vi "Address2ControlPoint.vi"(10 "Address":string) -> (1 "Contol\nPoint\nSuffix":T1, 3 "ControlPoint":string)   [LabVIEW 2009]
uses:
  lib/NTCP Client/Control Point Suffix.ctl
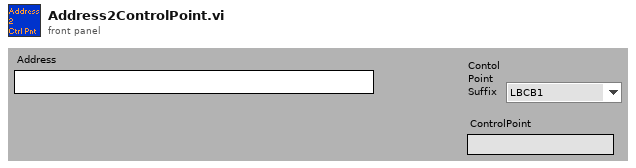
[diagram p1: front panel]
types:
  T1 = typedef "Control Point Suffix.ctl" = enum16{"LBCB1", "LBCB2", "ExternalSensors"}
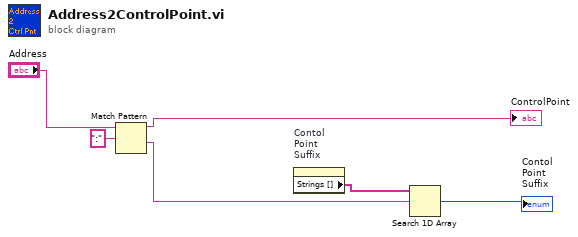
[diagram p0: block diagram]
diagram:
  n1 = Match Pattern(string="Address", regular expression=":") -> (before substring=→"ControlPoint":string, after substring=w2:string)  [unwired: 3 out]
  n2 = property on="Contol\nPoint\nSuffix" class="Enum (strict)"() -> ("Strings []"=w3:string[])  [unwired: 2 in, 2 out]
  n3 = Search 1D Array(1D array=w3, element=w2) -> (index of element=→"Contol\nPoint\nSuffix":i32)  [unwired: 1 out]
